vi "Update State.vi"(8 "error in (no error)":errorcluster, 10 "samples generated":i32, 11 "signal configuration":refnum<class "SV Signal.lvclass">) -> (0 "error out":errorcluster, 1 "segment done":bool, 2 "generation done":bool, 3 "signal configuration":refnum<class "SV Signal.lvclass">, 4 "measurement done":bool)   [LabVIEW 2017, in "SV Signal.lvclass"]
uses:
  <vilib>/addons/_NISVFA/_Generation/Signal Generation/SV Signal/SV Signal.lvclass
  <vilib>/addons/_NISVFA/_Generation/Signal Generation/SV Signal/sv_Signal State Attribute.ctl
  <vilib>/addons/_NISVFA/_Generation/Signal Generation/SV Signal/SV Signal.lvclass/SV Signal.ctl
  <vilib>/addons/_NISVFA/_Generation/Signal Generation/SV Signal/sv_Generation State.ctl
  <vilib>/addons/_NISVFA/_Generation/Signal Generation/SV Signal/sv_System Timing Model.ctl
  <vilib>/addons/_NISVFA/_Generation/subVIs/sv_Optimum Location.ctl
  <vilib>/addons/_NISVFA/_Generation/SoundVib_Generation.lvlib
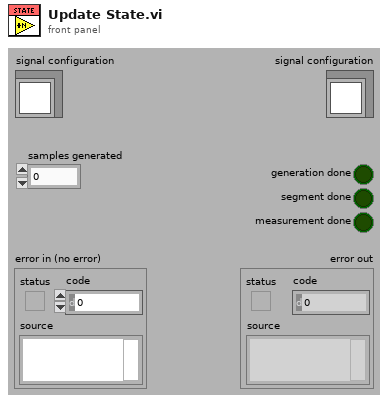
[diagram p1: front panel]
types:
  T1 = typedef "SV Signal.lvclass/sv_Signal State Attribute.ctl" = string
  T2 = typedef "SV Signal.lvclass/sv_Generation State.ctl" = enum16{"Idle", "Ramp Up", "Pre-Measurement Settling", "Measurement", "Post-Measurement Settling", "Discrete Sweep Transition", "Ramp Down", "Update"}
  T3 = typedef "SoundVib_Generation.lvlib/sv_Optimum Location.ctl" = enum16{"Zero Crossing, First Available", "Zero Crossing, Positive Slope", "Zero Crossing, Negative Slope", "Peak or Valley", "Peak", "Valley"}
  T4 = typedef "SV Signal.lvclass/sv_System Timing Model.ctl" = i64
  T5 = cluster{"system timing model":T4, "state":cluster{"RESET":bool, "generator timestamp":timestamp, "elapsed seconds":dbl, "elapsed samples":u64, "generation state":T2, "time offset at state":dbl, "samples generated at state":u64, "signal state":variant}, "duration of state":dbl, "samples remaining at state":i32}
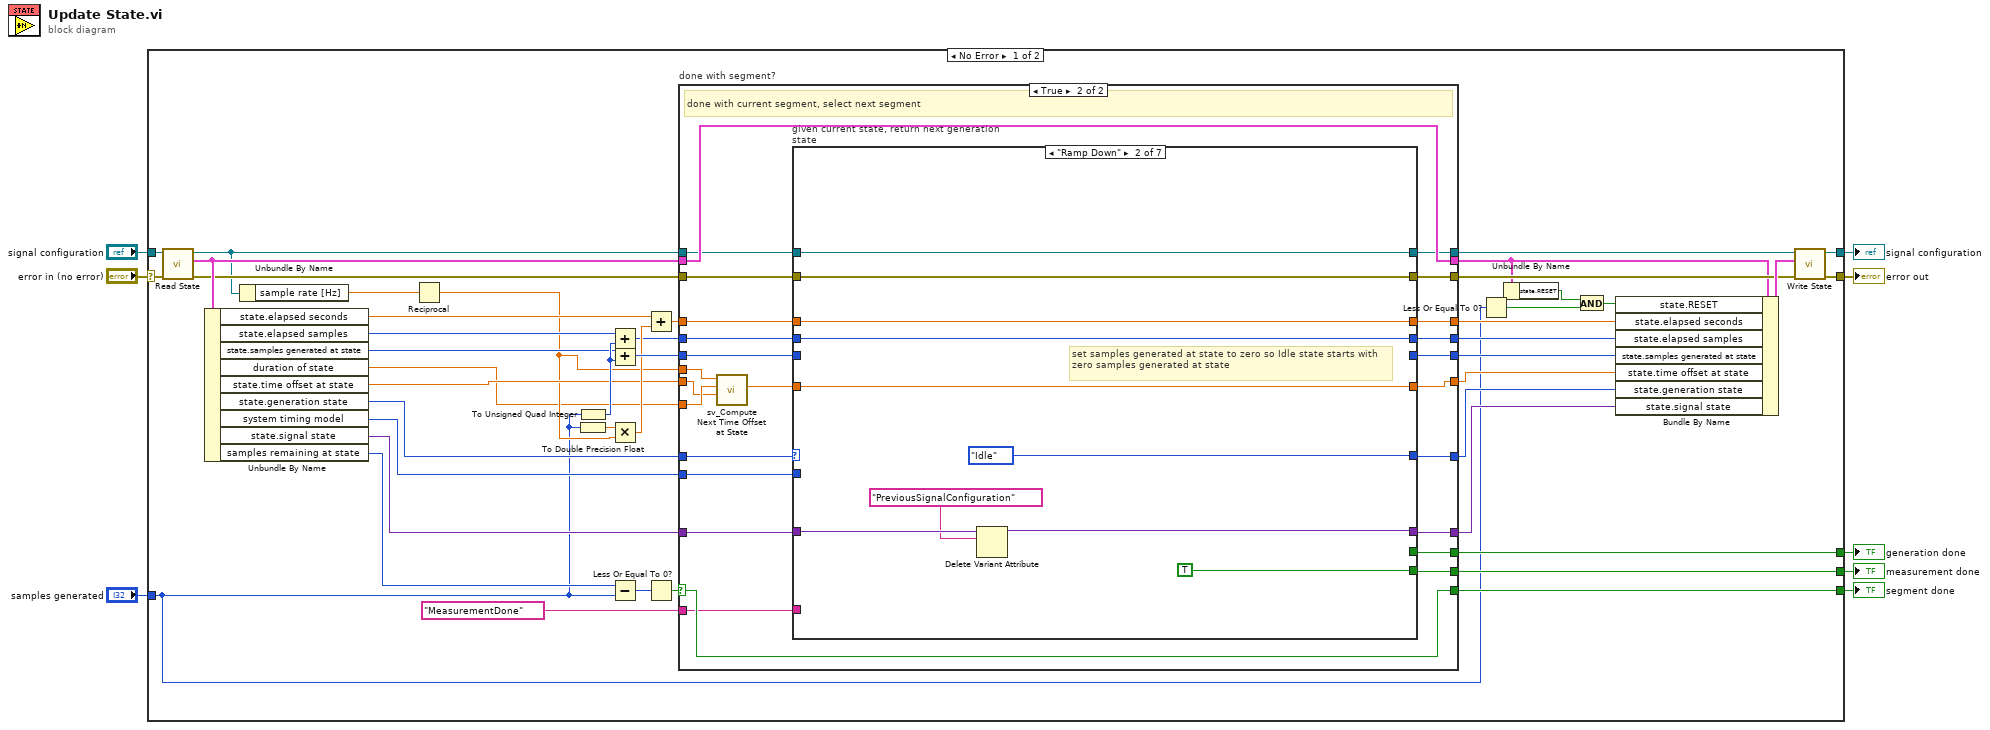
[diagram p0: block diagram]
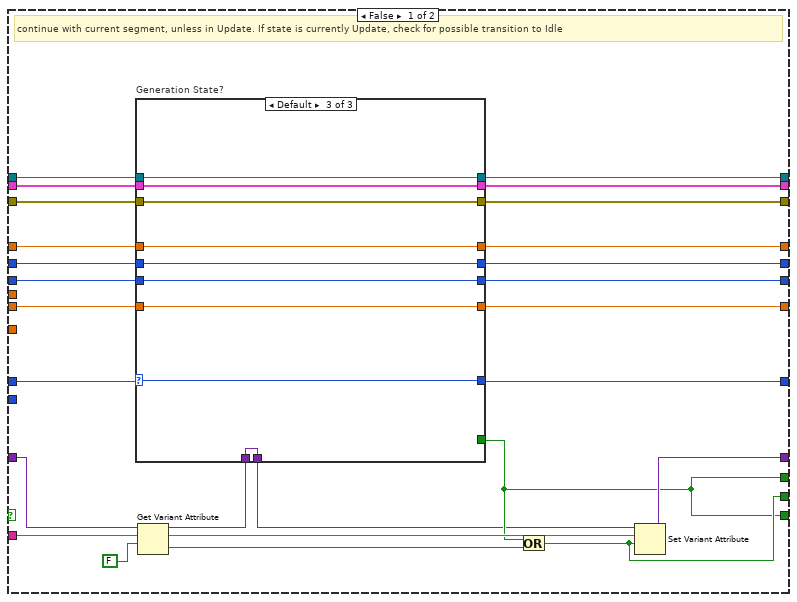
[diagram p2: hidden frame]
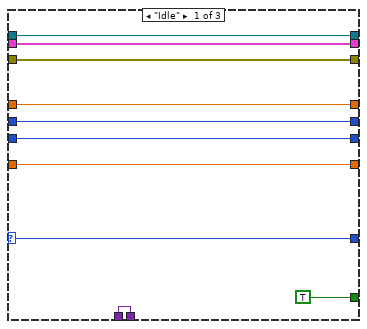
[diagram p3: hidden frame]
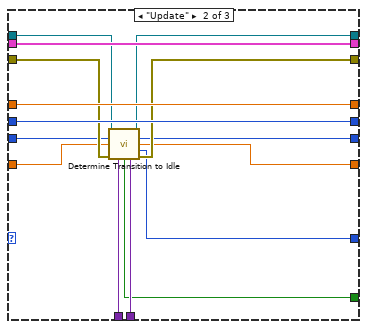
[diagram p4: hidden frame]
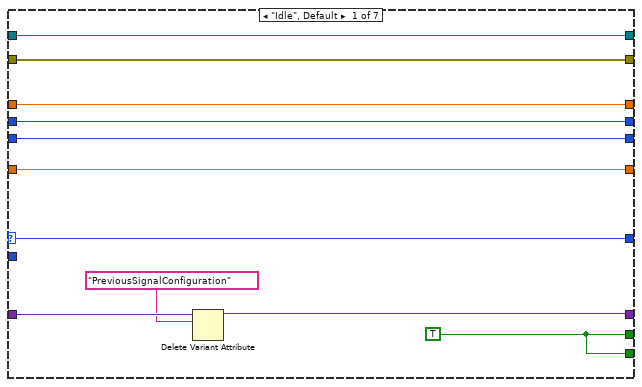
[diagram p5: hidden frame]
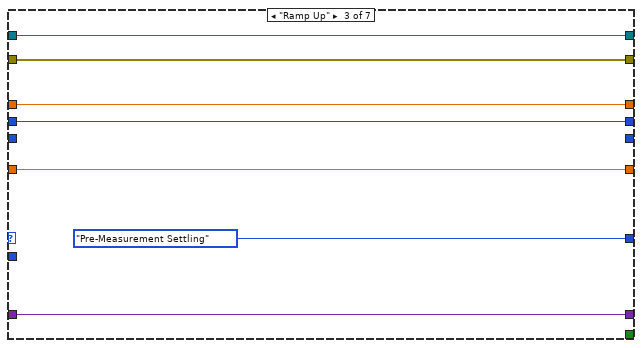
[diagram p6: hidden frame]
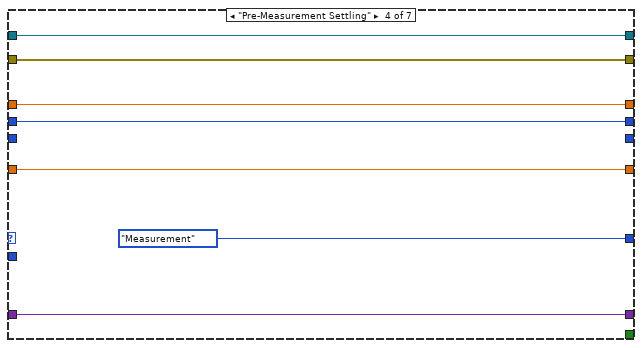
[diagram p7: hidden frame]
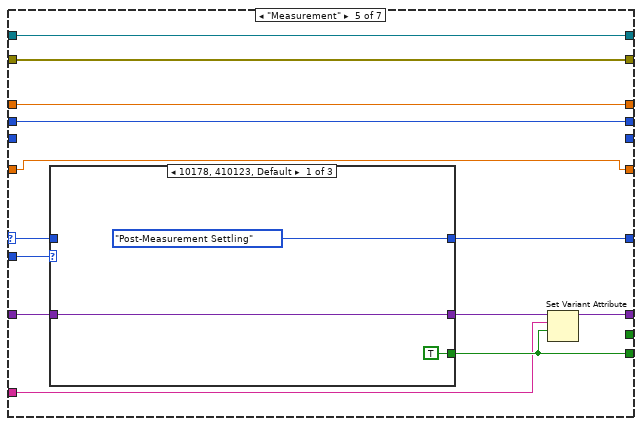
[diagram p8: hidden frame]
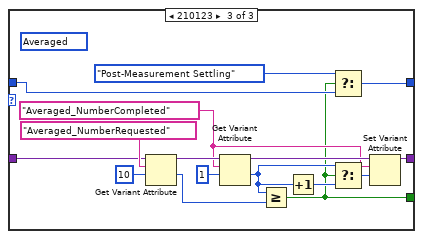
[diagram p10: hidden frame]
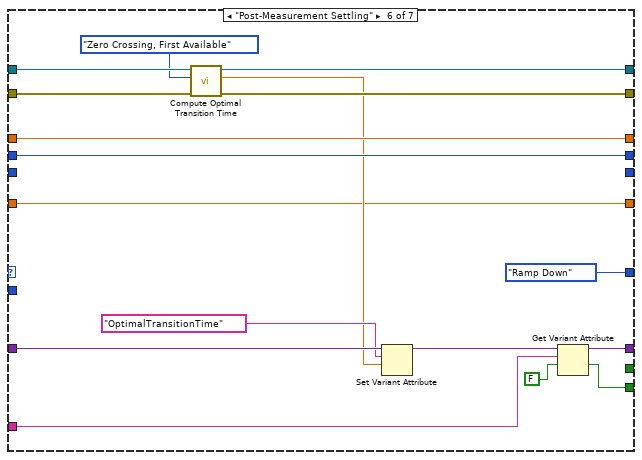
[diagram p11: hidden frame]
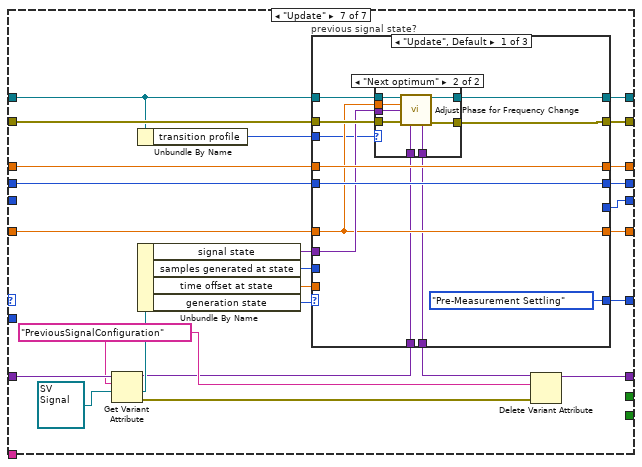
[diagram p12: hidden frame]
diagram:
  n1 = case shown="No Error" "error in (no error)" {
    selector: "error in (no error)" -> [w39 w286]
    tunnel: [w38 w286] -> w7
    tunnel: [w40 w287] -> w5
    tunnel: "signal configuration" -> [w43 w287]
    tunnel: "samples generated" -> [w9 _]
    tunnel: [w20 _] -> w3
    tunnel: [w44 _] -> w2
    tunnel: [w19 _] -> w1
    frame No Error {
      n2 = call <vilib>:"Read State.vi"("error in (no error)"=w39, "signal configuration"=w43) -> ("error out"=w29:errorcluster, "generator state"=w30:T5, "signal configuration"=w22:refnum<class "SV Signal.lvclass">)  [unwired: 7 in]
      n3 = Unbundle By Name(w30) -> ("state.elapsed seconds"=w47:dbl, "state.elapsed samples"=w52:u64, "state.samples generated at state"=w36:u64, "duration of state"=w15:dbl, "state.time offset at state"=w17:dbl, "state.generation state"=w46:T2, "system timing model"=w45:T4, "state.signal state"=w33:variant, "samples remaining at state"=w21:i32)
      n4 = Unbundle By Name(w22) -> ("sample rate [Hz]"=w42:dbl)
      n5 = Reciprocal(x=w42) -> (1/x=w16:dbl)
      n6 = To Unsigned Quad Integer(1:w9) -> (0:w37:u64)
      n7 = To Double Precision Float(number=w9) -> (double precision float=w51:dbl)
      n8 = Add(x=w52, y=w37) -> (x+y=w27:u64)
      n9 = Add(x=w36, y=w37) -> (x+y=w35:u64)
      n10 = Multiply(x=w51, y=w16) -> (x*y=w34:dbl)
      n11 = Subtract(x=w21, y=w9) -> (x-y=w49:i32)
      n12 = Add(x=w47, y=w34) -> (x+y=w25:dbl)
      n13 = Less Or Equal To 0?(x=w49) -> (x <= 0?=w50:bool)
      n14 = case "done with segment?" shown="True" w50 {
        selector: w50 -> [_ w132]
        tunnel: [w53 w136] -> w32
        tunnel: w45 -> [_ w135]
        tunnel: w46 -> [w71 w134]
        tunnel: [w66 w133] -> w20
        tunnel: [w70 w118] -> w14
        tunnel: [w68 w117] -> w48
        tunnel: [w66 w132] -> w44
        tunnel: w35 -> [w69 w112]
        tunnel: w17 -> [w67 w113]
        tunnel: w33 -> [w77 w131]
        tunnel: [w76 w130] -> w31
        tunnel: w22 -> [w64 w128]
        tunnel: w30 -> [w62 w129]
        tunnel: w29 -> [w60 w126]
        tunnel: [w57 w122] -> w28
        tunnel: w27 -> [w56 w121]
        tunnel: [w59 w124] -> w26
        tunnel: w25 -> [w58 w123]
        tunnel: [w65 w127] -> w24
        tunnel: [w63 w129] -> w13
        tunnel: [w61 w125] -> w23
        tunnel: [w72 w120] -> w19
        tunnel: T1 "MeasurementDone" ("name") -> [w75 w119]
        tunnel: w16 -> [_ w115]
        tunnel: w15 -> [_ w114]
        frame False {
          # "continue with current segment, unless in Update. If state is currently Update, check for possible transition to Idle"
          n15 = Get Variant Attribute(Variant=w77, name=w75, default value (empty Variant)=FALSE) -> (duplicate Variant=w55:variant, value=w73:bool)  [unwired: 1 in, 2 out]
          n16 = case "Generation State?" shown="Default" w71 {
            selector: w71 -> [w78 _ w103]
            tunnel: [w87 w93 w111] -> w70
            tunnel: w69 -> [w87 w95 w111]
            tunnel: [w86 w92 w110] -> w68
            tunnel: w67 -> [w86 w94 w110]
            tunnel: [TRUE w88 _] -> w66
            tunnel: [w84 w98 w109] -> w65
            tunnel: w64 -> [w84 w99 w109]
            tunnel: [w83 w102 w108] -> w63
            tunnel: w62 -> [w83 w102 w108]
            tunnel: [w82 w96 w107] -> w61
            tunnel: w60 -> [w82 w97 w107]
            tunnel: [w81 w101 w106] -> w59
            tunnel: w58 -> [w81 w101 w106]
            tunnel: [w80 w100 w105] -> w57
            tunnel: w56 -> [w80 w100 w105]
            tunnel: w55 -> [w79 w91 w104]
            tunnel: [w79 w90 w104] -> w54
            tunnel: [w78 w89 w103] -> w53
            frame "Idle" {
            }
            frame "Update" {
              n17 = call <vilib>:"Determine Transition to Idle.vi"("SV Signal in"=w99, "samples generated at state in"=w95, "time offset at state in"=w94, "error in (no error)"=w97, "signal state in"=w91) -> ("SV Signal out"=w98:refnum<class "SV Signal.lvclass">, "samples generated at state out"=w93:u64, "time offset at state out"=w92:dbl, "generation state out"=w89:T2, "transitioned to Idle?"=w88:bool, "signal state out"=w90:variant, "error out"=w96:errorcluster)  [unwired: 4 in]
            }
            frame Default {
            }
          }
          n18 = Or(x=w66, y=w73) -> (x .or. y?=w72:bool)
          n19 = Set Variant Attribute(Variant=w54, name=w75, value=w72) -> (Variant out=w76:variant)  [unwired: 1 in, 2 out]
        }
        frame True {
          # "done with current segment, select next segment"
          n20 = call <vilib>:"sv_Compute Next Time Offset at State.vi"("time offset at previous state"=w113, "duration of previous state"=w114, "dt"=w115) -> ("time offset at next state"=w116:dbl)  [unwired: 8 in]
          n21 = case "given current state, return next generation state" shown="\"Ramp Down\"" w134 {
            selector: w134 -> [w138 _ _ _ w177 _ _]
            tunnel: w135 -> [_ _ _ _ w183 _ _]
            tunnel: [w138 sv_Generation_State."Idle" ("generation state") sv_Generation_State."Pre-Measurement Settling" ("generation state") sv_Generation_State."Measurement" ("generation state") w184 sv_Generation_State."Ramp Down" ("generation state") w240] -> w136
            tunnel: [w143 _ _ _ _ _ _] -> w133
            tunnel: w131 -> [w142 w152 w163 w170 w182 w210 w246]
            tunnel: [w141 w151 w163 w170 w175 w219 w247] -> w130
            tunnel: w128 -> [w147 w156 w162 w169 w181 w215 w224]
            tunnel: [w147 w156 w162 w169 w181 w213 w234] -> w127
            tunnel: w126 -> [w146 w155 w161 w168 w180 w214 w232]
            tunnel: [w146 w155 w161 w168 w180 w212 w233] -> w125
            tunnel: [w145 w154 w160 w167 w179 w221 w231] -> w124
            tunnel: w123 -> [w145 w154 w160 w167 w179 w221 w230]
            tunnel: [w144 w153 w159 w166 w178 w220 w229] -> w122
            tunnel: w121 -> [w144 w153 w159 w166 w178 w220 w228]
            tunnel: [w143 TRUE ("found") _ _ w174 w216 _] -> w120
            tunnel: w119 -> [_ _ _ _ w173 w218 _]
            tunnel: [w137 _ _ _ _ _ w239] -> w118
            tunnel: [w139 w149 w158 w165 w172 w206 w236] -> w117
            tunnel: w116 -> [w139 w149 w158 w165 w172 w206 w235]
            tunnel: w112 -> [w137 _ _ _ _ _ _]
            frame "Idle", Default {
              w143 = TRUE
              n22 = Delete Variant Attribute(6:T1 "PreviousSignalConfiguration" ("name (all attributes)"), 7:w142) -> (3:w141:variant)  [unwired: 1 in, 2 out]
            }
            frame "Ramp Down" {
              # "set samples generated at state to zero so Idle state starts with zero samples generated at state"
              n23 = Delete Variant Attribute(6:T1 "PreviousSignalConfiguration" ("name (all attributes)"), 7:w152) -> (3:w151:variant)  [unwired: 1 in, 2 out]
            }
            frame "Ramp Up" {
            }
            frame "Pre-Measurement Settling" {
            }
            frame "Measurement" {
              n24 = case shown="10178, 410123, Default" w183 {
                tunnel: [sv_Generation_State."Post-Measurement Settling" ("generation state") w188 w196] -> w184
                tunnel: [w186 w189 w197] -> w176
                tunnel: w182 -> [w186 w189 w198]
                tunnel: w177 -> [_ w188 w195]
                tunnel: [TRUE _ w190] -> w174
                frame 10178, 410123, Default {
                }
                frame 10123, 110123 {
                }
                frame 210123 {
                  w191 = T1 "Averaged_NumberCompleted" ("name")
                  (unwired) T4 210123 items=["Finite"=10178, "-"=-1, "Continuous"=10123, "-"=-2, "Settled"=110123, "Averaged"=210123, "Discrete Sweep"=310123, "Continuous Sweep"=410123] ("system timing model")
                  n25 = Get Variant Attribute(Variant=w198, name=T1 "Averaged_NumberRequested", default value (empty Variant)=10 ("samples generated")) -> (duplicate Variant=w204:variant, value=w202:i32)  [unwired: 1 in, 2 out]
                  n26 = Get Variant Attribute(Variant=w204, name=w191, default value (empty Variant)=1 ("samples generated")) -> (duplicate Variant=w205:variant, value=w193:i32)  [unwired: 1 in, 2 out]
                  n27 = Greater Or Equal?(x=w193, y=w202) -> (x >= y?=w190:bool)
                  n28 = Increment(x=w193) -> (x+1=w194:i32)
                  n29 = Select(t=sv_Generation_State."Post-Measurement Settling" ("generation state"), s=w190, f=w195) -> (s? t:f=w196:T2)
                  n30 = Select(t=w193, s=w190, f=w194) -> (s? t:f=w192:i32)
                  n31 = Set Variant Attribute(Variant=w205, name=w191, value=w192) -> (Variant out=w197:variant)  [unwired: 1 in, 2 out]
                }
              }
              n32 = Set Variant Attribute(Variant=w176, name=w173, value=w174) -> (Variant out=w175:variant)  [unwired: 1 in, 2 out]
            }
            frame "Post-Measurement Settling" {
              n33 = call-dynamic "Compute Optimal Transition Time.vi"("error in (no error)"=w214, "optimum"=sv_Optimum_Location."Zero Crossing, First Available", "SV Signal in"=w215) -> ("error out"=w212:errorcluster, "optimal transition time"=w207:dbl, "SV Signal out"=w213:refnum<class "SV Signal.lvclass">)  [unwired: 6 in]
              n34 = Set Variant Attribute(Variant=w210, name=T1 "OptimalTransitionTime" ("attribute"), value=w207) -> (Variant out=w209:variant)  [unwired: 1 in, 2 out]
              n35 = Get Variant Attribute(Variant=w209, name=w218, default value (empty Variant)=FALSE ("found")) -> (duplicate Variant=w219:variant, value=w216:bool)  [unwired: 1 in, 2 out]
            }
            frame "Update" {
              w244 = T1 "PreviousSignalConfiguration" ("name (all attributes)")
              n36 = Get Variant Attribute(Variant=w246, name=w244, default value (empty Variant)=refnum<class "SV Signal.lvclass"> refnum ("signal configuration")) -> (duplicate Variant=w226:variant, value=w242:refnum<class "SV Signal.lvclass">, error out=w243:errorcluster)  [unwired: 1 in, 1 out]
              n37 = Unbundle By Name(w224) -> ("transition profile"=w223:enum16{"Immediate", "Next optimum", "Ramp"})
              n38 = Unbundle By Name(w242) -> ("signal state"=w227:variant, "samples generated at state"=w237:u64, "time offset at state"=w238:dbl, "generation state"=w241:T2)
              n39 = case "previous signal state?" shown="\"Update\", Default" w241 {
                selector: w241 -> [_ w278 w285]
                tunnel: [sv_Generation_State."Pre-Measurement Settling" ("generation state") w278 w285] -> w240
                tunnel: [_ w277 _] -> w239
                tunnel: w238 -> [_ w276 _]
                tunnel: w237 -> [_ w277 _]
                tunnel: [w251 w276 w284] -> w236
                tunnel: w235 -> [w251 _ w284]
                tunnel: [w255 w272 w280] -> w234
                tunnel: w224 -> [w256 w272 w280]
                tunnel: [w253 w273 w281] -> w233
                tunnel: w232 -> [w254 w273 w281]
                tunnel: [w258 w274 w282] -> w231
                tunnel: w230 -> [w258 w274 w282]
                tunnel: [w257 w275 w283] -> w229
                tunnel: w228 -> [w257 w275 w283]
                tunnel: w227 -> [w252 _ _]
                tunnel: w226 -> [w250 w271 w279]
                tunnel: [w249 w271 w279] -> w225
                tunnel: w223 -> [w248 _ _]
                frame "Update", Default {
                  n40 = case shown="\"Next optimum\"" w248 {
                    tunnel: w256 -> [w262 w270]
                    tunnel: [w262 w269] -> w255
                    tunnel: w254 -> [w261 w268]
                    tunnel: [w261 w267] -> w253
                    tunnel: w252 -> [_ w266]
                    tunnel: w251 -> [_ w265]
                    tunnel: w250 -> [w260 w264]
                    tunnel: [w260 w263] -> w249
                    frame "Immediate", Default {
                    }
                    frame "Next optimum" {
                      n41 = call <vilib>:"Adjust Phase for Frequency Change.vi"("SV Signal in"=w270, "time offset at state"=w265, "previous signal state"=w266, "error in (no error)"=w268, "signal state in"=w264) -> ("SV Signal out"=w269:refnum<class "SV Signal.lvclass">, "signal state out"=w263:variant, "error out"=w267:errorcluster)  [unwired: 8 in]
                    }
                  }
                }
                frame "Ramp Down" {
                }
                frame "Idle" {
                }
              }
              n42 = Delete Variant Attribute(4:w243, 6:w244, 7:w225) -> (3:w247:variant)  [unwired: 2 out]
            }
          }
        }
      }
      n43 = Less Or Equal To 0?(x=w9) -> (x <= 0?=w11:bool)
      n44 = Unbundle By Name(w13) -> ("state.RESET"=w12:bool)
      n45 = And(x=w12, y=w11) -> (x .and. y?=w10:bool)
      n46 = Bundle By Name(cluster=w13, "state.RESET"=w10, "state.elapsed seconds"=w26, "state.elapsed samples"=w28, "state.samples generated at state"=w14, "state.time offset at state"=w48, "state.generation state"=w32, "state.signal state"=w31) -> (w41:T5)
      n47 = call <vilib>:"Write State.vi"("error in (no error)"=w23, "generator state"=w41, "signal configuration"=w24) -> ("error out"=w38:errorcluster, "signal configuration"=w40:refnum<class "SV Signal.lvclass">)  [unwired: 7 in]
    }
    frame Error {
    }
  }
  "error out" <- w7
  "signal configuration" <- w5
  "generation done" <- w3
  "segment done" <- w2
  "measurement done" <- w1
